vi "ExtractValue.vi"(2 "Filter 2":string, 3 "Filter 1":string, 4 "Input String":string) -> (0 "Output String":string, 1 "Output Number":dbl)   [LabVIEW 2021]
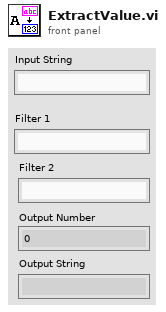
[diagram p1: front panel]
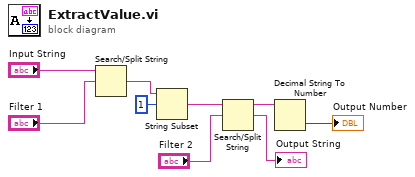
[diagram p0: block diagram]
diagram:
  n1 = Search/Split String(string="Input String", search string/char (-)="Filter 1") -> (match + rest of string=w6:string)  [unwired: 1 in, 2 out]
  n2 = String Subset(string=w6, offset (0)=1) -> (substring=w5:string)  [unwired: 1 in]
  n3 = Search/Split String(string=w5, search string/char (-)="Filter 2") -> (substring before match=w3:string, match + rest of string=→"Output String":string)  [unwired: 1 in, 1 out]
  n4 = Decimal String To Number(string=w3) -> (number=→"Output Number":i32)  [unwired: 2 in, 1 out]
